vi "Autonomous Independent.vi"   [LabVIEW 2019]
doc: "This VI is called when autonomous begins, and will automatically be terminated when autonomous ends. You can carry out timed or sensor driven robot movement independently without needing to return to the caller."
uses:
  Motion_Profiler_Class-master/MotionProfiles.lvclass
  <vilib>/Rock Robotics/WPI/ThirdParty/Phoenix-LabVIEW/Motor Controller/Sensor/CTRE_Phoenix_MotorControl_SetIntegratedSensorPosition_TalonFX.vi
  <vilib>/Rock Robotics/Network Tables/NT Read String.vi
  <vilib>/Utility/file.llb/Read Delimited Spreadsheet (string).vi
  <vilib>/Utility/file.llb/Read Delimited Spreadsheet (DBL).vi
panel:
  # "Be sure to right-click and choose Data Operations>>Make Current Value default if you want to save the array values with the VI"
types:
  T1 = typedef "WPI_MotorControlDeviceRef.ctl" = cluster{"DeviceStatus":errorcluster, "Type":T2, "PWM":cluster{"PWM Channel":T3, "DeadBand":T4}, "CAN":cluster{"Device Number":u8, "SetOutput VI Ref":variant, "GetOutput VI Ref":variant, "Enable VI Ref":variant, "Disable VI Ref":variant, "Data":variant}, "Invert":bool, "DIO PWM":cluster{"PWM \"Enable\" Channel":T3, "DIOChannel":T5, "PWM Rate":dbl}}
  T2 = typedef "WPI_MotorControlType.ctl" = enum16{"PWM", "CAN", "DIO PWM"}
  T3 = typedef "FPGA_DIOPWMChannel.ctl" = enum8{"PWM 0", "PWM 1", "PWM 2", "PWM 3", "PWM 4", "PWM 5", "PWM 6", "PWM 7", "PWM 8", "PWM 9", "PWM MXP 0", "PWM MXP 1", "PWM MXP 2", "PWM MXP 3", "PWM MXP 4", "PWM MXP 5", "PWM MXP 6", "PWM MXP 7", "PWM MXP 8", "PWM MXP 9", "Invalid"}
  T4 = typedef "WPI_PWMDeadband.ctl" = cluster{"Name":string, "maxPositivePwm":i32, "minPositivePwm":i32, "centerPwm":i32, "maxNegativePwm":i32, "minNegativePwm":i32, "angularRange":u16}
  T5 = typedef "FPGA_DIOChannel.ctl" = enum8{"DIO 0", "DIO 1", "DIO 2", "DIO 3", "DIO 4", "DIO 5", "DIO 6", "DIO 7", "DIO 8", "DIO 9", "DIO MXP 0", "DIO MXP 1", "DIO MXP 2", "DIO MXP 3", "DIO MXP 4", "DIO MXP 5", "DIO MXP 6", "DIO MXP 7", "DIO MXP 8", "DIO MXP 9", "DIO MXP 10", "DIO MXP 11", "DIO MXP 12", "DIO MXP 13", "DIO MXP 14", "DIO MXP 15", "SPI Port CS1", "SPI Port CS2", "SPI Port CS3", "SPI Port MISO", "SPI Port MOSI", "Invalid"}
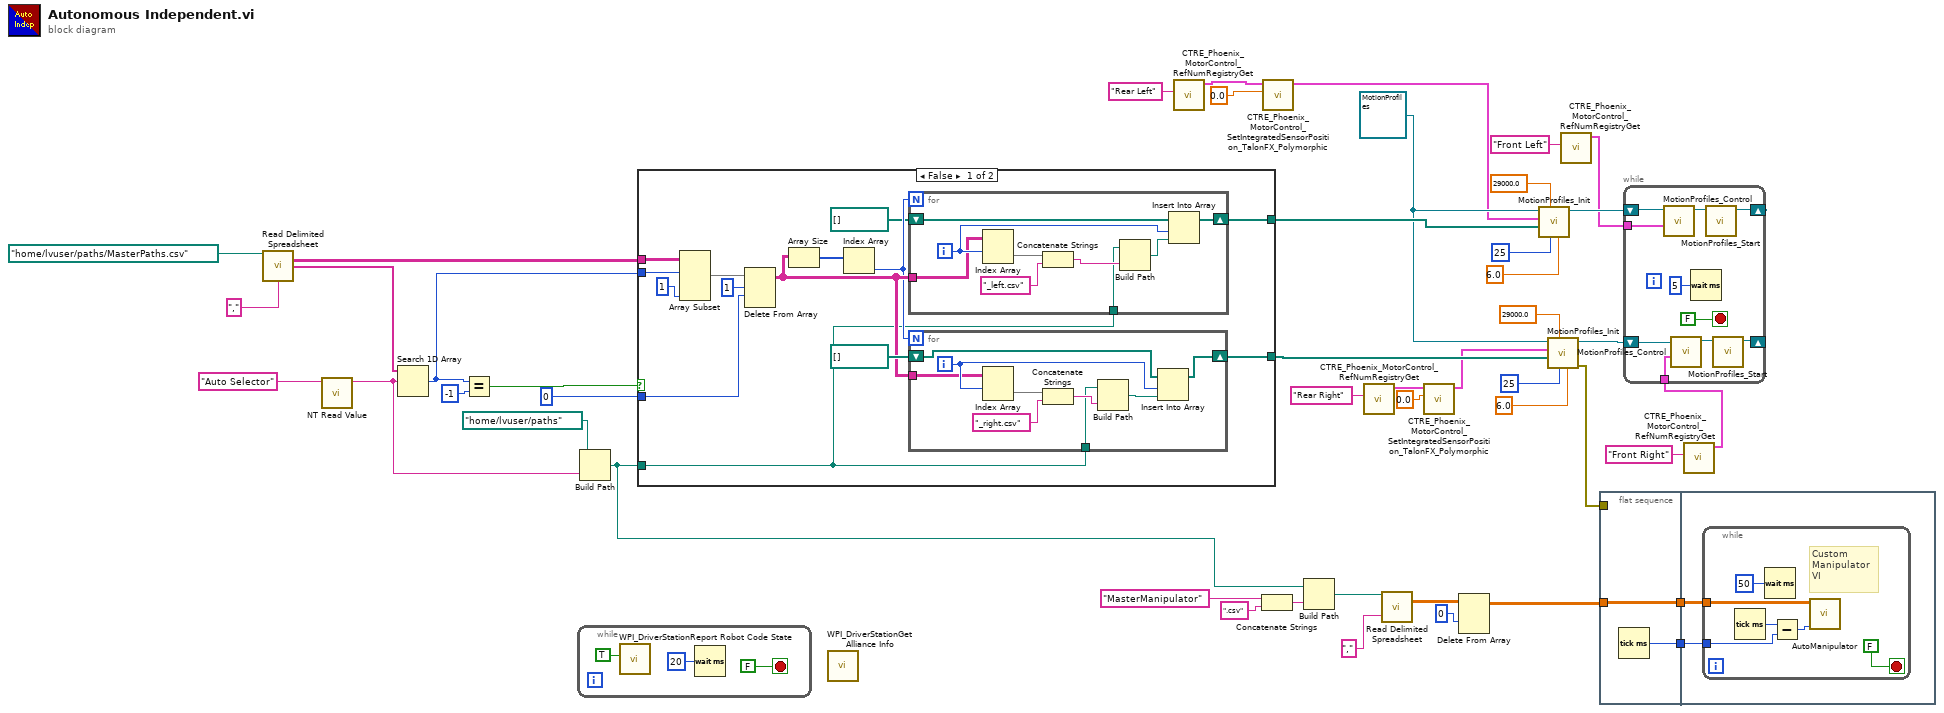
[diagram p0: block diagram]
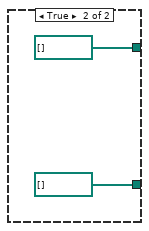
[diagram p2: hidden frame]
diagram:
  w22 = refnum<class "MotionProfiles.lvclass"> refnum ("MotionProfiles.lvclass")
  n1 = call-poly <vilib>:"Read Delimited Spreadsheet.vi"("file path (dialog if empty)"=path "/home/lvuser/paths/MasterPaths.csv" ("file path (use dialog)"), "delimiter (\\t)"="," ("delimiter (\\t)")) -> ("all rows"=w33:string[][], "first row"=w36:string[])  [unwired: 8 in, 4 out]
  n2 = call-poly <vilib>:"NT Read Value.vi"("Name"="Auto Selector") -> ("String"=w5:string)  [unwired: 9 in, 1 out]
  n3 = Search 1D Array(1D array=w36, element=w5) -> (index of element=w32:i32)  [unwired: 1 in]
  n4 = Equal?(x=w32, y=-1) -> (x = y?=w34:bool)
  n5 = while {
    stop <- FALSE stop-if-true
    n6 = call <vilib>:"WPI_DriverStationReport Robot Code State.vi"("Autonomous"=TRUE) -> ()  [unwired: 10 in, 1 out]
    n7 = Wait (ms)(milliseconds to wait=u32 20) -> ()  [unwired: 1 out]
  }
  n8 = Build Path(base path=path "/home/lvuser/paths" ("file path (use dialog)"), name or relative path=w5) -> (appended path=w2:path)
  n9 = case shown="False" w34 {
    tunnel: w33 -> [w63 _]
    tunnel: w32 -> [w62 _]
    tunnel: [w56 path[] [] ("CSV File Path")] -> w27
    tunnel: [w52 path[] [] ("CSV File Path")] -> w23
    tunnel: w2 -> [w50 _]
    tunnel: 0 ("index (row)") -> [w51 _]
    frame False {
      n10 = Array Subset(array=w63, index (row)=w62, length (col)=1 ("length")) -> (w60:string[][])  [unwired: 2 in]
      n11 = Delete From Array(array=w60, length=1, index (row)=w51) -> (array with subset deleted=w55:string[][])  [unwired: 1 in, 1 out]
      n12 = Array Size(array=w55) -> (size(s)=w57:i32[])
      n13 = Index Array(array=w57) -> (element=w54:i32)  [unwired: 1 in]
      n14 = for {
        N: w54 -> [_]
        shift-right: [w71] -> w52
        shift-left: path[] [] ("CSV File Path") -> [w72]
        tunnel: w55 -> [w69]
        tunnel: w50 -> [w64]
        i -> [w70]
        n15 = Index Array(array=w69, index (row)=w70) -> (element=w68:string[])  [unwired: 1 in]
        n16 = Concatenate Strings(w68, "_left.csv" ("string")) -> (w66:string)
        n17 = Build Path(base path=w64, name or relative path=w66) -> (appended path=w65:path)
        n18 = Insert Into Array(array=w72, index=w70, new element=w65) -> (w71:path[])
      }
      n19 = for {
        N: w54 -> [_]
        shift-right: [w80] -> w56
        shift-left: path[] [] ("CSV File Path") -> [w81]
        tunnel: w55 -> [w78]
        tunnel: w50 -> [w73]
        i -> [w79]
        n20 = Index Array(array=w78, index (row)=w79) -> (element=w76:string[])  [unwired: 1 in]
        n21 = Concatenate Strings(w76, "_right.csv" ("string")) -> (w74:string)
        n22 = Build Path(base path=w73, name or relative path=w74) -> (appended path=w75:path)
        n23 = Insert Into Array(array=w81, index=w79, new element=w75) -> (w80:path[])
      }
    }
    frame True {
    }
  }
  n24 = call <vilib>:"WPI_DriverStationGet Alliance Info.vi"() -> ()  [unwired: 12 out]
  n25 = call <vilib>:"CTRE_Phoenix_MotorControl_RefNumRegistryGet.vi"("refnum name"="Rear Left") -> ("PhoenixMotorControlDevRef"=w41:T1)  [unwired: 9 in, 1 out]
  n26 = Concatenate Strings("MasterManipulator" ("string"), ".csv" ("string")) -> (w16:string)
  n27 = call-poly <vilib>:"CTRE_Phoenix_MotorControl_SetIntegratedSensorPosition_TalonFX_Polymorphic.vi"("New Position"=0.0, "PhoenixMotorControlDevRef"=w41) -> ("PhoenixMotorControlDevRef"=w8:T1)  [unwired: 8 in, 1 out]
  n28 = Build Path(base path=w2, name or relative path=w16) -> (appended path=w14:path)
  n29 = call <vilib>:"CTRE_Phoenix_MotorControl_RefNumRegistryGet.vi"("refnum name"="Rear Right") -> ("PhoenixMotorControlDevRef"=w39:T1)  [unwired: 9 in, 1 out]
  n30 = call-poly <vilib>:"Read Delimited Spreadsheet.vi"("file path (dialog if empty)"=w14, "delimiter (\\t)"="," ("delimiter (\\t)")) -> ("all rows"=w17:dbl[][])  [unwired: 8 in, 5 out]
  n31 = call-poly <vilib>:"CTRE_Phoenix_MotorControl_SetIntegratedSensorPosition_TalonFX_Polymorphic.vi"("New Position"=0.0, "PhoenixMotorControlDevRef"=w39) -> ("PhoenixMotorControlDevRef"=w9:T1)  [unwired: 8 in, 1 out]
  n32 = Delete From Array(array=w17, index (row)=0) -> (array with subset deleted=w13:dbl[][])  [unwired: 2 in, 1 out]
  n33 = call "MotionProfiles_Init.vi"("Wheel_Diameter (in)"=6.0, "MP_Frame_Rate_(ms)"=25, "Encoder_CPR_4x"=29000.0, "CSV File Path"=w23, "PhoenixMotorControlDevRef"=w8, "MotionProfiles in"=w22) -> ("MotionProfiles out"=w10:refnum<class "MotionProfiles.lvclass">)  [unwired: 4 in, 1 out]
  n34 = call "MotionProfiles_Init.vi"("Wheel_Diameter (in)"=6.0, "MP_Frame_Rate_(ms)"=25, "Encoder_CPR_4x"=29000.0, "CSV File Path"=w27, "PhoenixMotorControlDevRef"=w9, "MotionProfiles in"=w22) -> ("error out"=w12:errorcluster, "MotionProfiles out"=w11:refnum<class "MotionProfiles.lvclass">)  [unwired: 4 in]
  n35 = call <vilib>:"CTRE_Phoenix_MotorControl_RefNumRegistryGet.vi"("refnum name"="Front Left") -> ("PhoenixMotorControlDevRef"=w7:T1)  [unwired: 9 in, 1 out]
  n36 = flat-sequence {
    tunnel: [w85] -> w21
    tunnel: w13 -> [w84]
    tunnel: [w84] -> w20
    tunnel: w12 -> [_]
    tunnel: w21 -> [w87]
    tunnel: w20 -> [w86]
    frame #0 {
      n37 = Tick Count (ms)() -> (millisecond timer value=w85:u32)
    }
    frame #1 {
      n38 = while {
        tunnel: w87 -> [w91]
        tunnel: w86 -> [w88]
        stop <- FALSE stop-if-true
        # "Custom\nManipulator\nVI"
        n39 = Tick Count (ms)() -> (millisecond timer value=w92:u32)
        n40 = Wait (ms)(milliseconds to wait=u32 50) -> ()  [unwired: 1 out]
        n41 = Subtract(x=w92, y=w91) -> (x-y=w89:u32)
        n42 = call "AutoManipulator.vi"("Time"=w89, "array"=w88) -> ()  [unwired: 10 in]
      }
    }
  }
  n43 = call <vilib>:"CTRE_Phoenix_MotorControl_RefNumRegistryGet.vi"("refnum name"="Front Right") -> ("PhoenixMotorControlDevRef"=w6:T1)  [unwired: 9 in, 1 out]
  n44 = while {
    shift-right: [w99] -> _
    shift-left: w11 -> [w98]
    shift-right: [w97] -> _
    shift-left: w10 -> [w96]
    tunnel: w7 -> [w95]
    tunnel: w6 -> [w94]
    stop <- FALSE stop-if-true
    n45 = call "MotionProfiles_Control.vi"("PhoenixMotorControlDevRef Slave"=w95, "MotionProfiles in"=w96) -> ("MotionProfiles out"=w100:refnum<class "MotionProfiles.lvclass">)  [unwired: 8 in, 1 out]
    n46 = call "MotionProfiles_Control.vi"("PhoenixMotorControlDevRef Slave"=w94, "MotionProfiles in"=w98) -> ("MotionProfiles out"=w101:refnum<class "MotionProfiles.lvclass">)  [unwired: 8 in, 1 out]
    n47 = Wait (ms)(milliseconds to wait=u32 5) -> ()  [unwired: 1 out]
    n48 = call "MotionProfiles_Start.vi"("MotionProfiles in"=w100) -> ("MotionProfiles out"=w97:refnum<class "MotionProfiles.lvclass">)  [unwired: 9 in, 1 out]
    n49 = call "MotionProfiles_Start.vi"("MotionProfiles in"=w101) -> ("MotionProfiles out"=w99:refnum<class "MotionProfiles.lvclass">)  [unwired: 9 in, 1 out]
  }
